vi "Open FB.vi"(8 "error in (no error)":errorcluster caption="错误输入（无错误）", 11 "Nested in":refnum<class "UI Template with RefNums FBCtrl.lvclass">) -> (0 "error out":errorcluster caption="错误输出", 3 "Nested out":refnum<class "UI Template with RefNums FBCtrl.lvclass">)   [LabVIEW 2020, in "UI Template with RefNums FBCtrl.lvclass"]
uses:
  UI Template with RefNums FBCtrl.lvclass
  UI Template with RefNums FBCtrl.lvclass/UI Template with RefNums FBCtrl.ctl
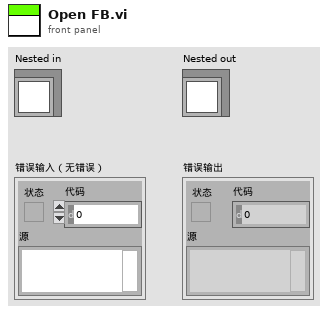
[diagram p1: front panel]
types:
  T1 = enum32{"Invalid", "Standard", "Closed", "Hidden", "Minimized", "Maximized"}
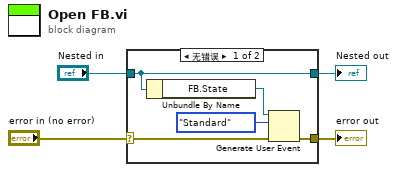
[diagram p0: block diagram]
diagram:
  n1 = case shown="无错误" "error in (no error)" {
    selector: "error in (no error)" -> [w8 w11]
    tunnel: [w7 w11] -> w3
    tunnel: [w9 w10] -> w1
    tunnel: "Nested in" -> [w9 w10]
    frame No Error {
      n2 = Unbundle By Name(w9) -> ("FB.State"=w6:refnum<user-event>)
      n3 = Generate User Event(user event=w6, event data cluster=T1."Standard" ("事件数据"), error in=w8) -> (error out=w7:errorcluster)  [unwired: 1 in, 1 out]
    }
    frame Error {
    }
  }
  "error out" <- w3
  "Nested out" <- w1
